vi "Motor_SetSpeed.vi"(8 "error in":errorcluster, 9 "Speed":dbl min=-1.0 max=1.0, 10 "PWM_Channel":T1=1 items=["Invalid"=0, "PWM1"=1, "PWM2"=2, "PWM9"=9, "PWM10"=10]) -> (0 "error out":errorcluster)   [LabVIEW 2009, in "Motor.lvlib"]
doc: "This VI is used to set speed of the motor. It requires the following inputs: \nPWM channel - channel to which the motor is connected; \nSpeed - speed value in range -1..+1. Here -1 corresponds to full reverse speed, +1 to full forward speed, 0 - stop the motor."
uses:
  Motor.lvlib
  PWM/PWM_Name.ctl
  ControllerType.ctl
  PWM.lvlib
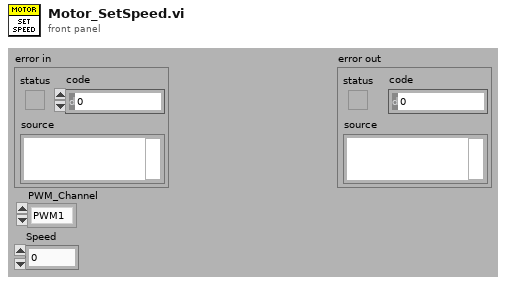
[diagram p1: front panel]
types:
  T1 = typedef "PWM.lvlib/PWM_Name.ctl" = u16
  T2 = typedef "Motor.lvlib/ControllerType.ctl" = u16
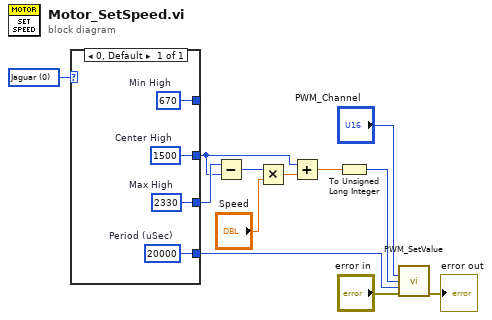
[diagram p0: block diagram]
diagram:
  w11 = T2 0 items=["Jaguar"] ("ControllerType")
  n1 = case shown="0, Default" w11 {
    tunnel: [w16] -> w4
    tunnel: [w15] -> _
    tunnel: [w14] -> w9
    tunnel: [w13] -> w10
    frame 0, Default {
      w13 = u32 2330  # Max High
      w14 = u32 1500  # Center High
      w15 = u32 670  # Min High
      w16 = u32 20000  # Period (uSec)
    }
  }
  n2 = Subtract(x=w10, y=w9) -> (x-y=w8:u32)
  n3 = Multiply(x=w8, y="Speed") -> (x*y=w6:dbl)
  n4 = Add(x=w9, y=w6) -> (x+y=w5:dbl)
  n5 = To Unsigned Long Integer(number=w5) -> (unsigned 32bit integer=w3:u32)
  n6 = call "PWM_SetValue.vi"("PWM"="PWM_Channel", "High (uSec)"=w3, "Period (uSec)"=w4, "error in"="error in") -> ("error out"=→"error out":errorcluster)  [unwired: 11 in]
